vi "EncoderValuesDashboard.vi"(1 "FrontRightReset":bool, 2 "FrontLeftReset":bool, 3 "ArmReset":bool, 4 "Teleop?":bool) -> (0 "ArmEncoderValues":i32)   [LabVIEW 2018]
uses:
  <vilib>/Rock Robotics/WPI/ThirdParty/Phoenix-LabVIEW/Motor Controller/Get/CTRE_Phoenix_MotorController_GetSelectedSensorData.vi
  <vilib>/Rock Robotics/Network Tables/NT Write Number.vi
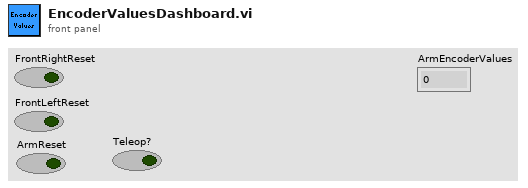
[diagram p1: front panel]
types:
  T1 = typedef "WPI_MotorControlDeviceRef.ctl" = cluster{"DeviceStatus":errorcluster, "Type":T2, "PWM":cluster{"PWM Channel":T3, "DeadBand":T4}, "CAN":cluster{"Device Number":u8, "SetOutput VI Ref":variant, "GetOutput VI Ref":variant, "Enable VI Ref":variant, "Disable VI Ref":variant, "Data":variant}, "Invert":bool, "DIO PWM":cluster{"PWM \"Enable\" Channel":T3, "DIOChannel":T5, "PWM Rate":dbl}}
  T2 = typedef "WPI_MotorControlType.ctl" = enum16{"PWM", "CAN", "DIO PWM"}
  T3 = typedef "FPGA_DIOPWMChannel.ctl" = enum8{"PWM 0", "PWM 1", "PWM 2", "PWM 3", "PWM 4", "PWM 5", "PWM 6", "PWM 7", "PWM 8", "PWM 9", "PWM MXP 0", "PWM MXP 1", "PWM MXP 2", "PWM MXP 3", "PWM MXP 4", "PWM MXP 5", "PWM MXP 6", "PWM MXP 7", "PWM MXP 8", "PWM MXP 9", "Invalid"}
  T4 = typedef "WPI_PWMDeadband.ctl" = cluster{"Name":string, "maxPositivePwm":i32, "minPositivePwm":i32, "centerPwm":i32, "maxNegativePwm":i32, "minNegativePwm":i32, "angularRange":u16}
  T5 = typedef "FPGA_DIOChannel.ctl" = enum8{"DIO 0", "DIO 1", "DIO 2", "DIO 3", "DIO 4", "DIO 5", "DIO 6", "DIO 7", "DIO 8", "DIO 9", "DIO MXP 0", "DIO MXP 1", "DIO MXP 2", "DIO MXP 3", "DIO MXP 4", "DIO MXP 5", "DIO MXP 6", "DIO MXP 7", "DIO MXP 8", "DIO MXP 9", "DIO MXP 10", "DIO MXP 11", "DIO MXP 12", "DIO MXP 13", "DIO MXP 14", "DIO MXP 15", "SPI Port CS1", "SPI Port CS2", "SPI Port CS3", "SPI Port MISO", "SPI Port MOSI", "Invalid"}
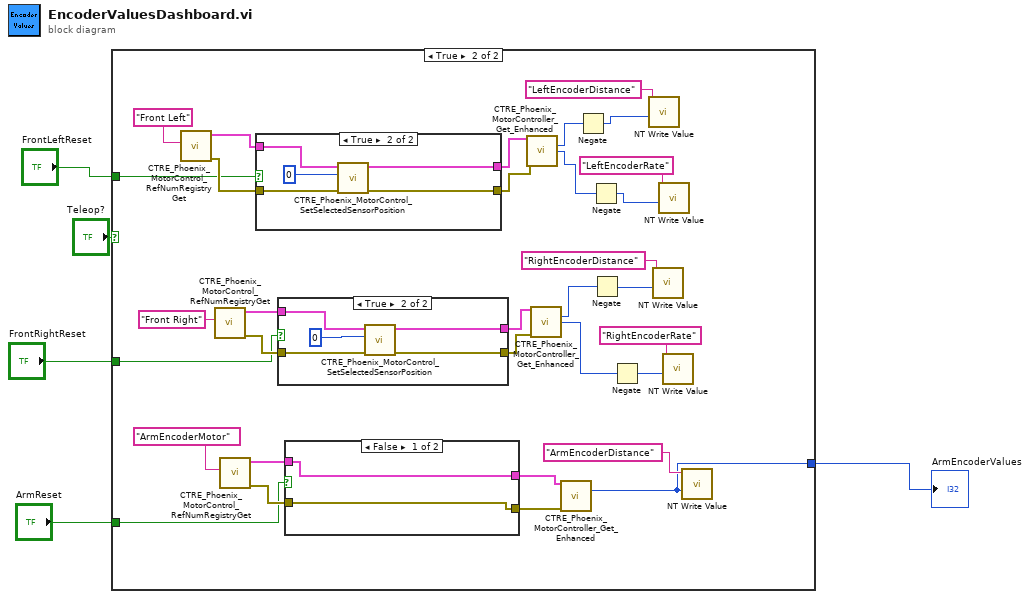
[diagram p0: block diagram]
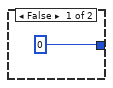
[diagram p2: hidden frame]
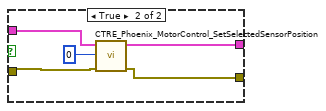
[diagram p3: hidden frame]
diagram:
  n1 = case shown="True" "Teleop?" {
    tunnel: "FrontRightReset" -> [_ w16]
    tunnel: "FrontLeftReset" -> [_ w15]
    tunnel: "ArmReset" -> [_ w8]
    tunnel: [0 w7] -> w1
    frame False {
    }
    frame True {
      n2 = call <vilib>:"CTRE_Phoenix_MotorControl_RefNumRegistryGet.vi"("refnum name"="Front Left") -> ("error out"=w21:errorcluster, "PhoenixMotorControlDevRef"=w24:T1)  [unwired: 9 in]
      n3 = call <vilib>:"CTRE_Phoenix_MotorControl_RefNumRegistryGet.vi"("refnum name"="Front Right") -> ("error out"=w17:errorcluster, "PhoenixMotorControlDevRef"=w20:T1)  [unwired: 9 in]
      n4 = call <vilib>:"CTRE_Phoenix_MotorControl_RefNumRegistryGet.vi"("refnum name"="ArmEncoderMotor") -> ("error out"=w12:errorcluster, "PhoenixMotorControlDevRef"=w13:T1)  [unwired: 9 in]
      n5 = case shown="True" w15 {
        tunnel: w24 -> [w54 w59]
        tunnel: [w54 w58] -> w23
        tunnel: [w53 w57] -> w22
        tunnel: w21 -> [w53 w56]
        frame False {
        }
        frame True {
          n6 = call <vilib>:"CTRE_Phoenix_MotorControl_SetSelectedSensorPosition.vi"("error in (no error)"=w56, "New Sensor Position"=0, "PhoenixMotorControlDevRef"=w59) -> ("error out"=w57:errorcluster, "PhoenixMotorControlDevRef"=w58:T1)  [unwired: 7 in]
        }
      }
      n7 = case shown="True" w16 {
        tunnel: w20 -> [w47 w52]
        tunnel: [w47 w51] -> w19
        tunnel: [w46 w50] -> w18
        tunnel: w17 -> [w46 w49]
        frame False {
        }
        frame True {
          n8 = call <vilib>:"CTRE_Phoenix_MotorControl_SetSelectedSensorPosition.vi"("error in (no error)"=w49, "New Sensor Position"=0, "PhoenixMotorControlDevRef"=w52) -> ("error out"=w50:errorcluster, "PhoenixMotorControlDevRef"=w51:T1)  [unwired: 7 in]
        }
      }
      n9 = case shown="False" w8 {
        tunnel: w13 -> [w40 w44]
        tunnel: w12 -> [w39 w43]
        tunnel: [w39 w42] -> w10
        tunnel: [w40 w41] -> w9
        frame False {
        }
        frame True {
          n10 = call <vilib>:"CTRE_Phoenix_MotorControl_SetSelectedSensorPosition.vi"("error in (no error)"=w43, "New Sensor Position"=0, "PhoenixMotorControlDevRef"=w44) -> ("error out"=w42:errorcluster, "PhoenixMotorControlDevRef"=w41:T1)  [unwired: 7 in]
        }
      }
      n11 = call-poly <vilib>:"CTRE_Phoenix_MotorController_Get_Enhanced.vi"("PhoenixMotorControlDevRef"=w23, "error in"=w22) -> ("Position (Raw Sensor Units)"=w32:i32, "Velocity (Raw Sensor Units per 100 ms)"=w29:i32)  [unwired: 10 in, 2 out]
      n12 = call-poly <vilib>:"CTRE_Phoenix_MotorController_Get_Enhanced.vi"("PhoenixMotorControlDevRef"=w19, "error in"=w18) -> ("Position (Raw Sensor Units)"=w25:i32, "Velocity (Raw Sensor Units per 100 ms)"=w28:i32)  [unwired: 10 in, 2 out]
      n13 = call-poly <vilib>:"CTRE_Phoenix_MotorController_Get_Enhanced.vi"("PhoenixMotorControlDevRef"=w9, "error in"=w10) -> ("Position (Raw Sensor Units)"=w7:i32)  [unwired: 10 in, 3 out]
      n14 = Negate(x=w32) -> (-x=w31:i32)
      n15 = Negate(x=w29) -> (-x=w30:i32)
      n16 = Negate(x=w25) -> (-x=w26:i32)
      n17 = Negate(x=w28) -> (-x=w27:i32)
      n18 = call-poly <vilib>:"NT Write Value.vi"("Numeric"=w31, "Name"="LeftEncoderDistance") -> ()  [unwired: 9 in, 1 out]
      n19 = call-poly <vilib>:"NT Write Value.vi"("Numeric"=w26, "Name"="RightEncoderDistance") -> ()  [unwired: 9 in, 1 out]
      n20 = call-poly <vilib>:"NT Write Value.vi"("Numeric"=w30, "Name"="LeftEncoderRate") -> ()  [unwired: 9 in, 1 out]
      n21 = call-poly <vilib>:"NT Write Value.vi"("Numeric"=w27, "Name"="RightEncoderRate") -> ()  [unwired: 9 in, 1 out]
      n22 = call-poly <vilib>:"NT Write Value.vi"("Numeric"=w7, "Name"="ArmEncoderDistance") -> ()  [unwired: 9 in, 1 out]
    }
  }
  "ArmEncoderValues" <- w1
